vi "CRYSet Custom Editor Front Panel.vi"(11 "VI Ref":refnum<vi> caption="Vi Ref") -> ()   [LabVIEW 2013]
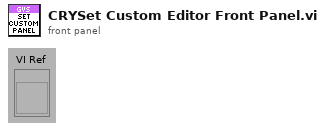
[diagram p1: front panel]
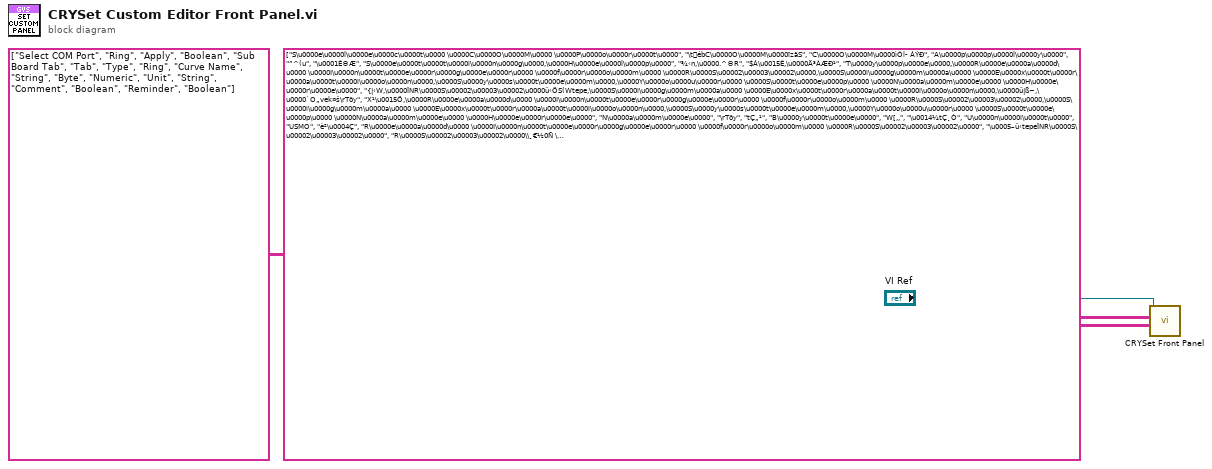
[diagram p0: block diagram]
diagram:
  n1 = call "CRYSet Front Panel.vi"("Caption(Boolean Text)"=string[][] [["S\u0000e\u0000l\u0000e\u0000c\u0000t\u0000 \u0000C\u0000O\u0000M\u0000 \u0000P\u0000o\u0000r\u0000t\u0000", "\tébC\u0000O\u0000M\u0000ïzãS", "C\u0000O\u0000M\u0000ìÓl­ ÁÝÐ"], ["A\u0000p\u0000p\u0000l\u0000y\u0000", "”^(u", "\u0001È©Æ"], ["S\u0000e\u0000t\u0000t\u0000i\u0000n\u0000g\u0000,\u0000H\u0000e\u0000l\u0000p\u0000", "¾‹n,\u0000.^©R", "$Á\u0015È,\u0000Ä³ÀÆÐ¹"], ["T\u0000y\u0000p\u0000e\u0000,\u0000R\u0000e\u0000a\u0000d\u0000 \u0000I\u0000n\u0000t\u0000e\u0000r\u0000g\u0000e\u0000r\u0000 \u0000f\u0000r\u0000o\u0000m\u0000 \u0000R\u0000S\u00002\u00003\u00002\u0000,\u0000S\u0000i\u0000g\u0000m\u0000a\u0000 \u0000E\u0000x\u0000t\u0000r\u0000a\u0000t\u0000i\u0000o\u0000n\u0000,\u0000S\u0000y\u0000s\u0000t\u0000e\u0000m\u0000,\u0000Y\u0000o\u0000u\u0000r\u0000 \u0000S\u0000t\u0000e\u0000p\u0000 \u0000N\u0000a\u0000m\u0000e\u0000 \u0000H\u0000e\u0000r\u0000e\u0000", "{|‹W,\u0000ÎNR\u0000S\u00002\u00003\u00002\u0000û‹ÖS(Wtepe,\u0000S\u0000i\u0000g\u0000m\u0000a\u0000 \u0000E\u0000x\u0000t\u0000r\u0000a\u0000t\u0000i\u0000o\u0000n\u0000,\u0000û|ß~,\u0000`O„vek¤š\rTðy", "X¹\u0015Ö,\u0000R\u0000e\u0000a\u0000d\u0000 \u0000I\u0000n\u0000t\u0000e\u0000r\u0000g\u0000e\u0000r\u0000 \u0000f\u0000r\u0000o\u0000m\u0000 \u0000R\u0000S\u00002\u00003\u00002\u0000,\u0000S\u0000i\u0000g\u0000m\u0000a\u0000 \u0000E\u0000x\u0000t\u0000r\u0000a\u0000t\u0000i\u0000o\u0000n\u0000,\u0000S\u0000y\u0000s\u0000t\u0000e\u0000m\u0000,\u0000Y\u0000o\u0000u\u0000r\u0000 \u0000S\u0000t\u0000e\u0000p\u0000 \u0000N\u0000a\u0000m\u0000e\u0000 \u0000H\u0000e\u0000r\u0000e\u0000"], ["N\u0000a\u0000m\u0000e\u0000", "\rTðy", "tÇ„¹"], ["B\u0000y\u0000t\u0000e\u0000", "W[‚‚", "\u0014¼tÇ¸Ò"], ["U\u0000n\u0000i\u0000t\u0000", "USMO", "è²\u0004Ç"], ["R\u0000e\u0000a\u0000d\u0000 \u0000I\u0000n\u0000t\u0000e\u0000r\u0000g\u0000e\u0000r\u0000 \u0000f\u0000r\u0000o\u0000m\u0000 \u0000R\u0000S\u00002\u00003\u00002\u0000", "\u0005–û‹tepeÎNR\u0000S\u00002\u00003\u00002\u0000", "R\u0000S\u00002\u00003\u00002\u0000\\¸€½0Ñ \u00009Æü­\u0018Â \u0000}Ç0®"], ["R\u0000e\u0000m\u0000i\u0000n\u0000d\u0000e\u0000r\u0000:\u0000 \u0000 \u0000Y\u0000o\u0000u\u0000 \u0000m\u0000u\u0000s\u0000t\u0000 \u0000e\u0000d\u0000i\u0000t\u0000 \u0000t\u0000h\u0000i\u0000s\u0000 \u0000c\u0000u\u0000s\u0000t\u0000o\u0000m\u0000 \u0000s\u0000t\u0000e\u0000p\u0000 \u0000f\u0000r\u0000o\u0000m\u0000\n\u0000w\u0000i\u0000t\u0000h\u0000i\u0000n\u0000 \u0000a\u0000 \u0000s\u0000e\u0000q\u0000u\u0000e\u0000n\u0000c\u0000e\u0000 \u0000f\u0000o\u0000r\u0000 \u0000i\u0000t\u0000 \u0000t\u0000o\u0000 \u0000r\u0000e\u0000m\u0000e\u0000m\u0000b\u0000e\u0000r\u0000 \u0000y\u0000o\u0000u\u0000r\u0000 \u0000s\u0000e\u0000t\u0000t\u0000i\u0000n\u0000g\u0000s\u0000.\u0000", "Ðc\u001aÿ`OÅ_{\u0016Ù*Nê[INek¤\n\u0000(W\u0000N*N^\u0017R-N\fÿ[°OO¨`v¾n\u0000\u0000", "LÅ¼¹:\u0000 \u0000$Á\u0015ÈDÇ \u0000ô¼tÈXÕ0®\u0004ÇXÕìÅ \u0000ü¬\u001cÈ,¸ÐÅ\u001cÁ \u0000\n\u0000tÇ \u0000¬¹©ÆÇ\u0015ÈXÇü¬\u001cÈmÕ©ºDÇ \u0000¸ÓÑÉXÕìÅ|ÅiÕÈ²ä².\u0000"]], "Control ID and Type(Label Name, Type)"=string[][] [["Select COM Port", "Ring"], ["Apply", "Boolean"], ["Sub Board Tab", "Tab"], ["Type", "Ring"], ["Curve Name", "String"], ["Byte", "Numeric"], ["Unit", "String"], ["Comment", "Boolean"], ["Reminder", "Boolean"]], "Vi Ref"="VI Ref") -> ()  [unwired: 9 in]
